vi "DLOS.vi"() -> ()   [LabVIEW 2015]
uses:
  scope/Agilent_546XX_Series/Agilent 546XX Series.lvlib
panel:
  in  "Scope Channel 2 Data":path
  in  "Scope Channel 1 Data":path
  in  "Trigger Delay":dbl
  in  "Time Range (sec/div)":dbl=0.0001 format="%#_13g"
  in  "Tigger Level (Volts)":dbl
  in  "Trigger Channel":u32(slide)=1 scale=1.0..2.0
  in  "Trigger Coupling":u32(slide) scale=0.0..1.0
  in  "Trigger Sweep Mode":string(combo)="Normal"
  in  "Capture Mode":string(combo)="Run"
  in  "Voltage Range (Channel 2)":dbl=1.0 format="%#_13g"
  in  "Voltage Range (Channel 1)":dbl=1.0 format="%#_13g"
  in  "VISA Scope":refnum<visa-resource-name>
  in  "VISA Boonton":refnum<visa-resource-name>
  in  "VISA Laser Trigger":refnum<visa-resource-name>
  in  "Stop":bool
  out "Laser Fire":bool
  in  "Laser Trigger Delay":dbl
  in  "Scope Read Delay":dbl
  out "Scope Read":bool
  out "error out":errorcluster
  in  "error in (no error)":errorcluster
  # "Scope Setup"
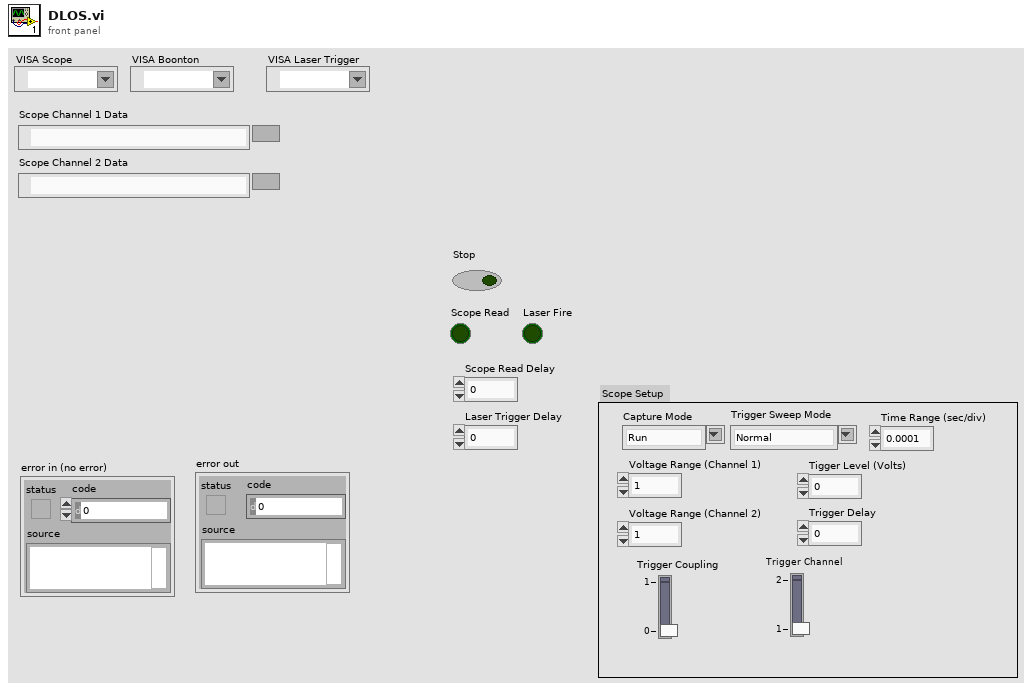
[diagram p1: front panel]
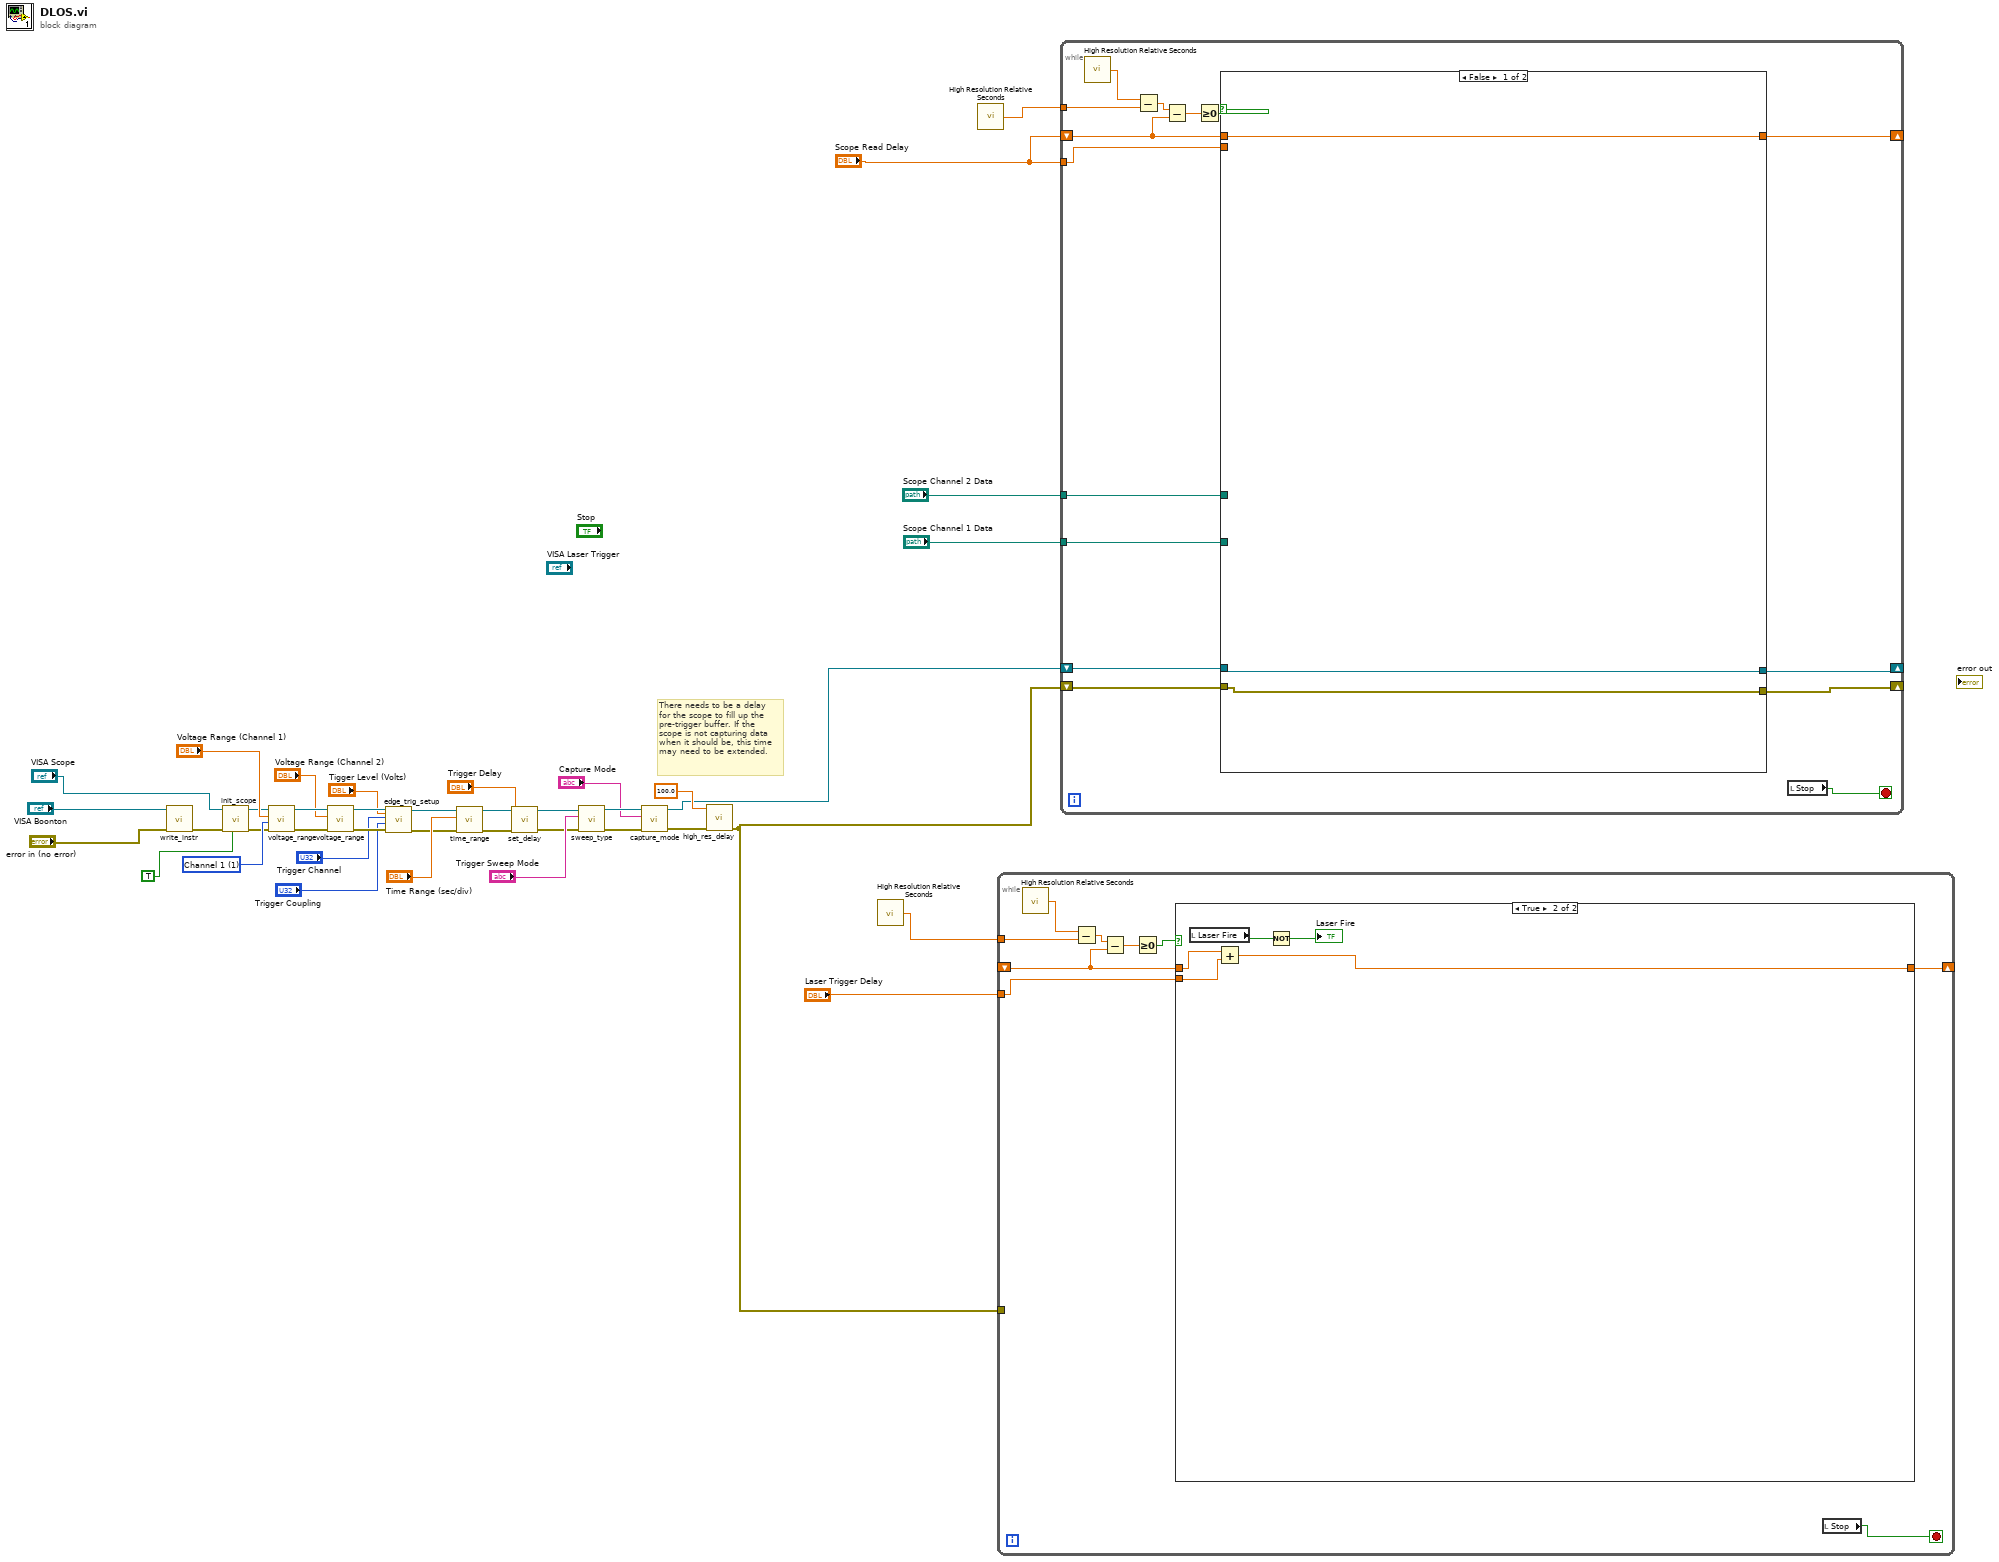
[diagram p0: block diagram]
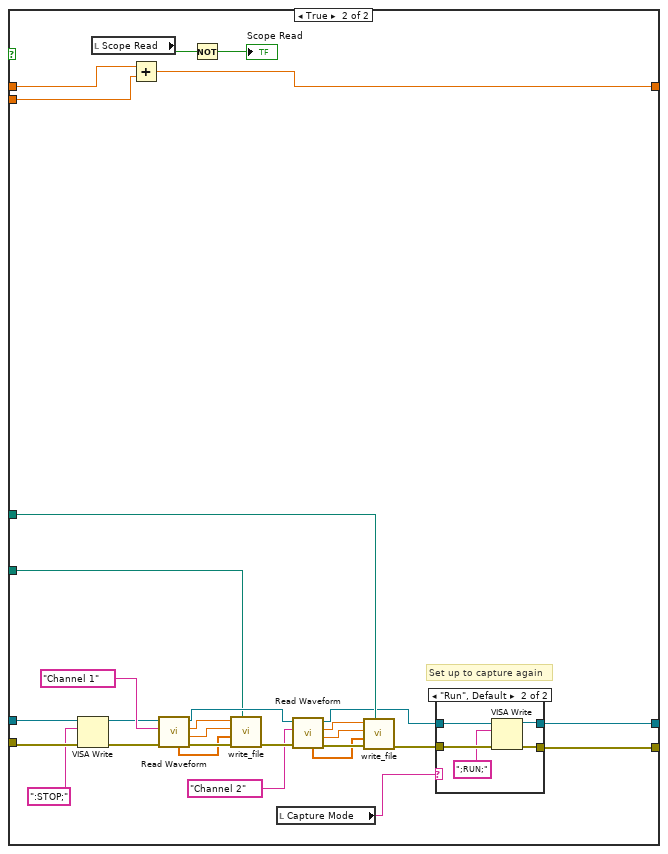
[diagram p3: hidden frame]
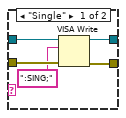
[diagram p4: hidden frame]
diagram:
  w32 = u32 1 items=["Channel 2"=2, "Channel 1"=1] ("Channel Select")
  # "There needs to be a delay\nfor the scope to fill up the\npre-trigger buffer. If the \nscope is not capturing data\nwhen it should be, this time\nmay need to be extended."
  n1 = call "write_instr.vi"("error in (no error)"="error in (no error)", "VISA In"="VISA Boonton") -> ("error out"=w8:errorcluster)  [unwired: 8 in, 1 out]
  n2 = call "init_scope.vi"("Autoscale initialization"=TRUE, "error in (no error)"=w8, "VISA Scope"="VISA Scope") -> ("error out"=w11:errorcluster, "VISA Scope Out"=w10:refnum<visa-resource-name>)  [unwired: 7 in]
  n3 = call "voltage_range.vi"("error in (no error)"=w11, "Channel Select"=w32, "Voltage"="Voltage Range (Channel 1)", "VISA In"=w10) -> ("error out"=w30:errorcluster, "VISA Out"=w31:refnum<visa-resource-name>)  [unwired: 6 in]
  n4 = call "voltage_range.vi"("error in (no error)"=w30, "Voltage"="Voltage Range (Channel 2)", "VISA In"=w31) -> ("error out"=w26:errorcluster, "VISA Out"=w27:refnum<visa-resource-name>)  [unwired: 7 in]
  n5 = call "edge_trig_setup.vi"("Tigger Level"="Tigger Level (Volts)", "error in (no error)"=w26, "Coupling"="Trigger Coupling", "Channel"="Trigger Channel", "VISA In"=w27) -> ("error out"=w20:errorcluster, "VISA Out"=w21:refnum<visa-resource-name>)  [unwired: 5 in]
  n6 = call "time_range.vi"("error in (no error)"=w20, "Time Range"="Time Range (sec/div)", "VISA In"=w21) -> ("error out"=w18:errorcluster, "VISA Out"=w19:refnum<visa-resource-name>)  [unwired: 7 in]
  n7 = call "set_delay.vi"("error in (no error)"=w18, "Delay"="Trigger Delay", "VISA Scope In"=w19) -> ("error out"=w15:errorcluster, "VISA Out"=w16:refnum<visa-resource-name>)  [unwired: 7 in]
  n8 = call "sweep_type.vi"("error in (no error)"=w15, "Sweep Type"="Trigger Sweep Mode", "VISA In"=w16) -> ("error out"=w13:errorcluster, "VISA Out"=w14:refnum<visa-resource-name>)  [unwired: 7 in]
  n9 = call "capture_mode.vi"("error in (no error)"=w13, "Capture Mode"="Capture Mode", "VISA In"=w14) -> ("error out"=w6:errorcluster, "VISA Out"=w3:refnum<visa-resource-name>)  [unwired: 7 in]
  n10 = call "high_res_delay.vi"("error in (no error)"=w6, "Delay (sec)"=100.0) -> ("error out"=w4:errorcluster)  [unwired: 9 in]
  n11 = call <vilib>:"High Resolution Relative Seconds.vi"() -> ("relative seconds"=w36:dbl)
  n12 = call <vilib>:"High Resolution Relative Seconds.vi"() -> ("relative seconds"=w39:dbl)
  n13 = while {
    tunnel: w36 -> [w48]
    shift-right: [w44] -> _
    shift-left: _ -> [w45]
    tunnel: "Laser Trigger Delay" -> [w41]
    tunnel: w4 -> [_]
    stop <- w40 stop-if-true
    n14 = call <vilib>:"High Resolution Relative Seconds.vi"() -> ("relative seconds"=w43:dbl)
    n15 = Subtract(x=w43, y=w48) -> (x-y=w42:dbl)
    n16 = Subtract(x=w42, y=w45) -> (x-y=w47:dbl)
    n17 = Greater Or Equal To 0?(x=w47) -> (x >= 0?=w46:bool)
    n18 = case shown="True" w46 {
      tunnel: [w49 w54] -> w44
      tunnel: w45 -> [w49 w52]
      tunnel: w41 -> [_ w51]
      frame False {
      }
      frame True {
        n19 = local read "Laser Fire"() -> (w53:bool)
        n20 = Add(x=w52, y=w51) -> (x+y=w54:dbl)
        n21 = Not(x=w53) -> (.not. x?=→"Laser Fire":bool)
      }
    }
    n22 = local read "Stop"() -> (w40:bool)
  }
  n23 = while {
    tunnel: w39 -> [w69]
    shift-right: [w65] -> _
    shift-left: "Scope Read Delay" -> [w66]
    tunnel: "Scope Read Delay" -> [w62]
    tunnel: "Scope Channel 1 Data" -> [w58]
    tunnel: "Scope Channel 2 Data" -> [w57]
    shift-right: [w55] -> _
    shift-left: w4 -> [w59]
    shift-right: [w56] -> _
    shift-left: w3 -> [w60]
    stop <- w61 stop-if-true
    n24 = call <vilib>:"High Resolution Relative Seconds.vi"() -> ("relative seconds"=w64:dbl)
    n25 = Subtract(x=w64, y=w69) -> (x-y=w63:dbl)
    n26 = Subtract(x=w63, y=w66) -> (x-y=w68:dbl)
    n27 = Greater Or Equal To 0?(x=w68) -> (x >= 0?=w67:bool)
    n28 = case shown="False" w67 {
      tunnel: [w72 w101] -> w65
      tunnel: w66 -> [w72 w98]
      tunnel: w62 -> [_ w97]
      tunnel: w60 -> [w71 w91]
      tunnel: w59 -> [w70 w90]
      tunnel: w58 -> [_ w83]
      tunnel: w57 -> [_ w78]
      tunnel: [w71 w74] -> w56
      tunnel: [w70 w73] -> w55
      frame False {
      }
      frame True {
        # "Set up to capture again"
        n29 = VISA Write(VISA resource name=w91, write buffer=":STOP;", error in (no error)=w90) -> (VISA resource name out=w87:refnum<visa-resource-name>, error out=w88:errorcluster)  [unwired: 1 out]
        n30 = local read "Scope Read"() -> (w99:bool)
        n31 = Add(x=w98, y=w97) -> (x+y=w101:dbl)
        n32 = call "Read Waveform.vi"("error in (no error)"=w88, "Channel"="Channel 1", "VISA Resource Name"=w87) -> ("error out"=w95:errorcluster, "x increment"=w93:dbl, "initial x"=w92:dbl, "VISA Resource Name Out"=w84:refnum<visa-resource-name>, "waveform array"=w94:dbl[])  [unwired: 3 in, 1 out]
        n33 = Not(x=w99) -> (.not. x?=→"Scope Read":bool)
        n34 = call "write_file.vi"("Data File"=w83, "error in (no error)"=w95, "Y Axis Data"=w94, "Step Size"=w93, "Initial Value"=w92) -> ("error out"=w86:errorcluster)  [unwired: 4 in, 1 out]
        n35 = local read "Capture Mode"() -> (w77:string)
        n36 = call "Read Waveform.vi"("error in (no error)"=w86, "Channel"="Channel 2", "VISA Resource Name"=w84) -> ("error out"=w82:errorcluster, "x increment"=w80:dbl, "initial x"=w79:dbl, "VISA Resource Name Out"=w75:refnum<visa-resource-name>, "waveform array"=w81:dbl[])  [unwired: 3 in, 1 out]
        n37 = call "write_file.vi"("Data File"=w78, "error in (no error)"=w82, "Y Axis Data"=w81, "Step Size"=w80, "Initial Value"=w79) -> ("error out"=w76:errorcluster)  [unwired: 4 in, 1 out]
        n38 = case shown="\"Run\", Default" w77 {
          tunnel: w76 -> [w106 w109]
          tunnel: w75 -> [w105 w108]
          tunnel: [w103 w111] -> w74
          tunnel: [w102 w110] -> w73
          frame "Single" {
            n39 = VISA Write(VISA resource name=w105, write buffer=":SING;", error in (no error)=w106) -> (VISA resource name out=w103:refnum<visa-resource-name>, error out=w102:errorcluster)  [unwired: 1 out]
          }
          frame "Run", Default {
            n40 = VISA Write(VISA resource name=w108, write buffer=";RUN;", error in (no error)=w109) -> (VISA resource name out=w111:refnum<visa-resource-name>, error out=w110:errorcluster)  [unwired: 1 out]
          }
        }
      }
    }
    n41 = local read "Stop"() -> (w61:bool)
  }
